vi "ElevatorSystemV2DriveToSetpoint.vi"(2 "Setpoints":dbl[](array[numeric]), 3 "Encoder Reading":dbl, 4 "Target Position":enum16{"Low", "High"}(ring)) -> (0 "Motor Output":dbl, 1 "Current Position":T1(ring))   [LabVIEW 2014]
panel:
  # "Low"
  # "High"
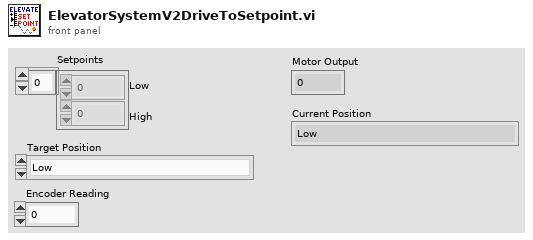
[diagram p1: front panel]
types:
  T1 = enum16{"Low", "High", "Intermediary (Between positions)"}
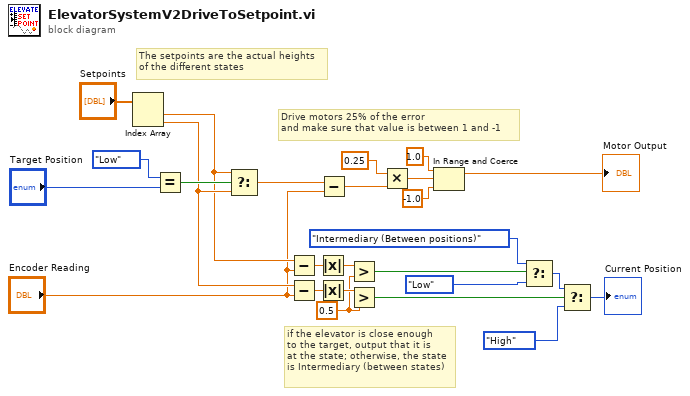
[diagram p0: block diagram]
diagram:
  w4 = 0.5 ("y")
  # "The setpoints are the actual heights\nof the different states"
  # "Drive motors 25% of the error\nand make sure that value is between 1 and -1"
  # "if the elevator is close enough\nto the target, output that it is\nat the state; otherwise, the state\nis Intermediary (between states)"
  n1 = Index Array(array="Setpoints") -> (element #1=w9:dbl, element #2=w16:dbl)  [unwired: 2 in]
  n2 = Equal?(x=enum16{"Low", "High"}."Low", y="Target Position") -> (x = y?=w24:bool)
  n3 = Select(t=w9, s=w24, f=w16) -> (s? t:f=w22:dbl)
  n4 = Subtract(x=w9, y="Encoder Reading") -> (x-y=w7:dbl)
  n5 = Subtract(x=w16, y="Encoder Reading") -> (x-y=w15:dbl)
  n6 = Absolute Value(x=w7) -> (abs(x)=w5:dbl)
  n7 = Absolute Value(x=w15) -> (abs(x)=w14:dbl)
  n8 = Subtract(x=w22, y="Encoder Reading") -> (x-y=w21:dbl)
  n9 = Greater?(x=w5, y=w4) -> (0:w6:bool)
  n10 = Greater?(x=w14, y=w4) -> (0:w13:bool)
  n11 = Multiply(x=0.25, y=w21) -> (x*y=w19:dbl)
  n12 = In Range and Coerce(upper limit=1.0, x=w19, lower limit=-1.0) -> (coerced(x)=→"Motor Output":dbl)  [unwired: 1 out]
  n13 = Select(t=T1."Intermediary (Between positions)" ("Current Position"), s=w6, f=T1."Low" ("Current Position")) -> (s? t:f=w10:T1)
  n14 = Select(t=w10, s=w13, f=T1."High" ("Current Position")) -> (s? t:f=→"Current Position":T1)
